vi "handleTitle.vi"(9 "类型":u16(ring) items=["直流", "交流"]) -> (0 "交流表头":string[](array[string]), 3 "直流表头":string[](array[string]))   [LabVIEW 2014]
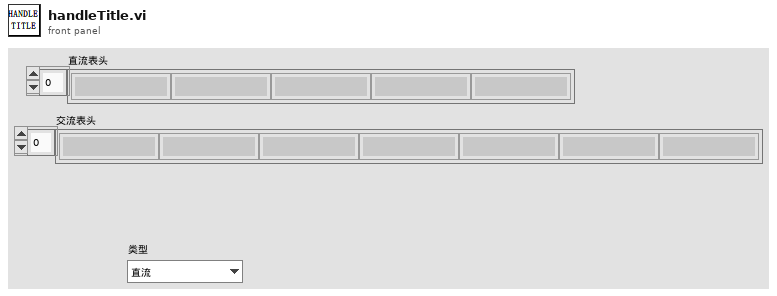
[diagram p1: front panel]
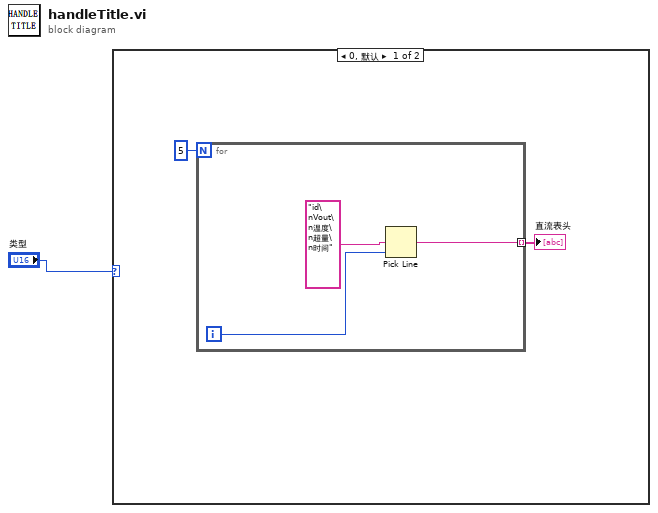
[diagram p0: block diagram]
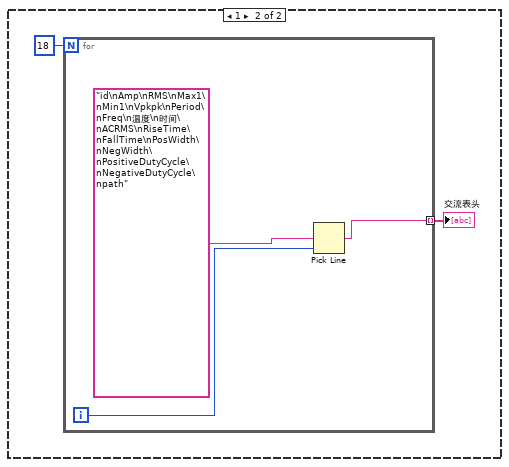
[diagram p2: hidden frame]
diagram:
  n1 = case shown="0, 默认" "类型" {
    frame 0, Default {
      n2 = for {
        N: 5 -> [_]
        tunnel: [w4] -> w3 mode=indexing
        i -> [w5]
        n3 = Pick Line(multi-line string="id\nVout\n温度\n超量\n时间", line index=w5) -> (output string=w4:string)  [unwired: 1 in]
      }
      "直流表头" <- w3
    }
    frame 1 {
      n4 = for {
        N: 18 -> [_]
        tunnel: [w9] -> w7 mode=indexing
        i -> [w10]
        n5 = Pick Line(multi-line string="id\nAmp\nRMS\nMax1\nMin1\nVpkpk\nPeriod\nFreq\n温度\n时间\nACRMS\nRiseTime\nFallTime\nPosWidth\nNegWidth\nPositiveDutyCycle\nNegativeDutyCycle\npath", line index=w10) -> (output string=w9:string)  [unwired: 1 in]
      }
      "交流表头" <- w7
    }
  }
